vi "3-4.vi"(2 "字符串 2":string, 3 "数值":dbl, 4 "字符串":string) -> (0 "数值 2":i32, 1 "字符串 3":string)   [LabVIEW 2017]
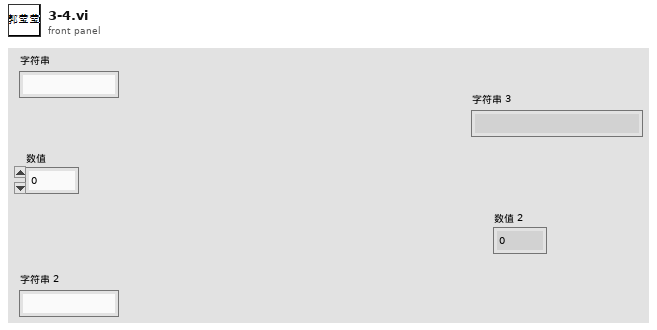
[diagram p1: front panel]
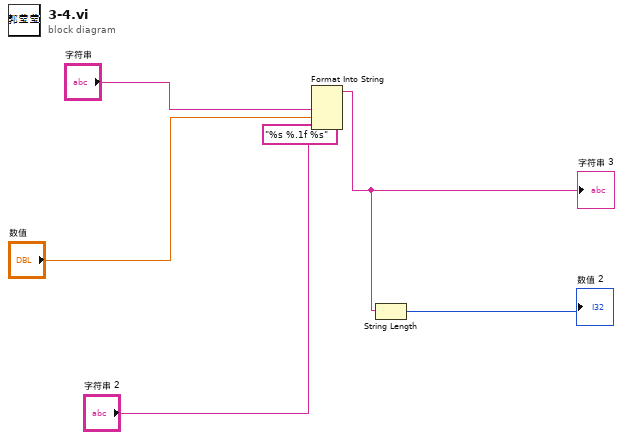
[diagram p0: block diagram]
diagram:
  n1 = Format Into String(format string="%s %.1f %s" ("格式字符串"), "字符串", "数值", "字符串 2") -> (resulting string=w3:string)  [unwired: 2 in, 1 out]
  "字符串 3" <- w3
  n2 = String Length(string=w3) -> (length=→"数值 2":i32)
